vi "UHR-Fleezers Control (host) -TL FB Corrected Ronen.vi"(0 "Tab Control":T5(tab)=enum."DAQ AI") -> ()   [LabVIEW 2013] (continued)
                    }
                  }
                }
                event Mouse Up {
                  n1349 = event-data() -> ("Button"=w2095:u16)  [unwired: 8 out]
                  n1350 = case shown="3" w2095 {
                    tunnel: [FALSE TRUE] -> w2096
                    frame 0, Default {
                    }
                    frame 3 {
                      n1351 = local write "Manipulating Trap"(FALSE ("Manipulating Trap")) -> ()
                    }
                  }
                }
              }
            }
          }
        }
      }
      event Mouse Move {
        n1352 = event-data() -> ()  [unwired: 6 out]
      }
    }
    n1353 = local read "Stop All"() -> (w1917:bool)
    n1354 = node-c288() -> ()  [unwired: 2 out]
  }
  n1355 = node-c288(w34) -> ()  [unwired: 1 out]
  n1356 = node-c288(w88) -> ()  [unwired: 1 out]
  n1357 = node-c288(w95) -> ()  [unwired: 1 out]
  n1358 = node-c288(i64 1 ("Period"), 1 ("Processor")) -> (w182:T25)  [unwired: 2 out]
  n1359 = timed-loop "Acquire Data" {
    tunnel: w44 -> [w2380]
    tunnel: w60 -> [w2379]
    tunnel: [w2410] -> w53
    tunnel: [w2404] -> w52
    timing: w182 -> [_]
    timing-out: [_] -> w181
    tunnel: w79 -> [w2215]
    stop <- "Stop All" stop-if-true
    (unwired) u32 0 ("Number of Elements")
    w2202 = "NI_ChannelName" ("name")
    n1360 = node-c288() -> ()  [unwired: 2 out]
    n1361 = First Call?() -> (First Call?: T/F=w2168:bool)
    n1362 = Or(x="Reset", y=w2168) -> (x .or. y?=w2169:bool)
    n1363 = local read "MCL Tracking"() -> (w2105:bool)
    n1364 = case "Reset data stream" shown="True" w2169 {
      tunnel: w2380 -> [w2478 w2486]
      tunnel: w2379 -> [w2477 w2485]
      tunnel: [w2478 w2480] -> w2103
      tunnel: [w2477 w2479] -> w2375
      frame False {
      }
      frame True {
        w2483 = TRUE ("AI to FIFO")
        n1365 = local write "Overflow (data lost)"(FALSE ("Overflow (data lost)")) -> ()
        n1366 = call "reset FPGA DMA.vi"("error in"=w2485, "FPGA VI Reference In"=w2486) -> ("error out"=w2481:errorcluster, "FPGA VI Reference Out"=w2482:T20)
        n1367 = xnode "Read/Write Control"("FPGA VI Reference In"=w2482, "error in"=w2481, "AI to FIFO"=w2483, "APD to FIFO"=w2483) -> ("FPGA VI Reference Out"=w2480:T20, "error out"=w2479:errorcluster)
      }
    }
    n1368 = Or(x="Start AOD Scan", y="Trap Raster Scan") -> (x .or. y?=w2331:bool)
    n1369 = case "Start AOM raster scan" shown="True" w2331 {
      tunnel: w2103 -> [w3215 w3225]
      tunnel: w2375 -> [w3214 w3224]
      tunnel: [w3215 w3218] -> w2102
      tunnel: [w3214 w3217] -> w2374
      frame False {
      }
      frame True {
        n1370 = case shown="True" "Restart DMA? (AOD)" {
          tunnel: [w3263 w3265] -> w3219
          tunnel: [w3262 w3264] -> w3220
          tunnel: w3225 -> [w3263 w3267]
          tunnel: w3224 -> [w3262 w3266]
          frame False {
          }
          frame True {
            n1371 = local write "Overflow (data lost)"(FALSE ("Overflow (data lost)")) -> ()
            n1372 = call "reset FPGA DMA.vi"("error in"=w3266, "FPGA VI Reference In"=w3267) -> ("error out"=w3264:errorcluster, "FPGA VI Reference Out"=w3265:T20)
          }
        }
        n1373 = local write "Trap Raster Scan"(FALSE ("Trap Raster Scan")) -> ()
        n1374 = case shown="True" "Move MCL Also?" {
          tunnel: w3220 -> [w3228 w3257]
          tunnel: w3219 -> [w3229 w3258]
          tunnel: [w3227 w3261] -> w3218
          tunnel: [w3226 w3260] -> w3217
          frame False {
            w3230 = TRUE ("AI to FIFO")
            n1375 = xnode "Read/Write Control"("FPGA VI Reference In"=w3229, "error in"=w3228, "AI to FIFO"=w3230, "APD to FIFO"=w3230, "Start scan"=w3230) -> ("FPGA VI Reference Out"=w3227:T20, "error out"=w3226:errorcluster)
          }
          frame True {
            w3254 = FALSE ("1D or 2D Scan?")
            w3259 = TRUE ("AI to FIFO")
            # "Count for MCL loop"
            # "N total cycles"
            # "N steps"
            # "V_int"
            n1376 = local read "Scan Range (nm)"() -> (w3236:dbl)
            n1377 = local read "Number of F/B Scans (AOD)"() -> (w3253:u16)
            n1378 = Sign(1:w3236) -> (0:w3235:dbl)
            n1379 = Compound Arithmetic op=MULTIPLY(w3236, "MCL Step Position Ratio", "MCL/AOM Scale Tweak") -> (w3240:dbl)
            n1380 = Negate(x=w3235) -> (-x=w3232:dbl)
            n1381 = Multiply(x=w3232, y="MCL Step Increment (V_int)") -> (x*y=w3234:dbl)
            n1382 = Divide(x=w3240, y="MCL X Cal (nm/V)") -> (x/y=w3246:dbl)
            n1383 = Multiply(x=32767.0 ("y"), y=w3246) -> (x*y=w3252:dbl)
            n1384 = local read "Total Counts (ticks)"() -> (w3237:u32)
            n1385 = local read "Cycles/step (AOD)"() -> (w3248:u64)
            n1386 = local read "Scan steps (AOD)"() -> (w3249:u64)
            n1387 = Divide(x=w3252, y=10.0) -> (x/y=w3245:dbl)
            n1388 = Divide(x=w3245, y="MCL Step Increment (V_int)") -> (x/y=w3243:dbl)
            n1389 = Absolute Value(x=w3243) -> (abs(x)=w3231:dbl)
            n1390 = Compound Arithmetic op=MULTIPLY(w3249, w3248, w3237) -> (w3244:u64)
            n1391 = local write "wait to reset values"(w3259) -> ()
            n1392 = local write "MCL Scanning"(w3259) -> ()
            n1393 = Divide(x=w3244, y=w3231) -> (x/y=w3241:dbl)
            "MCL Count" <- w3241
            n1394 = xnode "Read/Write Control"("FPGA VI Reference In"=w3258, "error in"=w3257, "Scan steps (MCL)"=w3231, "Number of scans (MCL)"=w3253, "Cycles per step (MCL)"=u64 1, "Scan freq.  increment (MCL)"=w3234, "1D or 2D Scan?"=w3254, "MCL Scan Axis"=w3254, "Cont. Scan (MCL)"=w3254, "MCL count"=w3241) -> ("FPGA VI Reference Out"=w3256:T20, "error out"=w3255:errorcluster)
            n1395 = xnode "Read/Write Control"("FPGA VI Reference In"=w3256, "error in"=w3255, "AI to FIFO"=w3259, "APD to FIFO"=w3259, "Start scan"=w3259, "Start scan (MCL)"=w3259) -> ("FPGA VI Reference Out"=w3261:T20, "error out"=w3260:errorcluster)
          }
        }
        "Raster Scanning..." <- TRUE ("Scanning...")
      }
    }
    n1396 = And(x="Save scans", y=w2331) -> (x .and. y?=w2373:bool)
    n1397 = Compound Arithmetic op=OR("Start MCL Scan", "Confocal Image", "Confocal Linescan") -> (w2329:bool)
    n1398 = And(x="Save Data (MCL)", y=w2329) -> (x .and. y?=w2372:bool)
    n1399 = case "Start MCL raster scan" shown="True" w2329 {
      tunnel: w2102 -> [w2769 w2784]
      tunnel: w2374 -> [w2768 w2783]
      tunnel: [w2769 w2779] -> w2138
      tunnel: [w2768 w2778] -> w2137
      tunnel: [FALSE w2777] -> w2358
      tunnel: "Start MCL Scan" -> [_ w2772]
      tunnel: "Confocal Image" -> [_ w2771]
      tunnel: "Confocal Linescan" -> [_ _]
      frame False {
      }
      frame True {
        w2777 = TRUE
        n1400 = case shown="True" "Restart DMA? (MCL)" {
          tunnel: [w2829 w2831] -> w2782
          tunnel: [w2828 w2830] -> w2781
          tunnel: w2784 -> [w2829 w2834]
          tunnel: w2783 -> [w2828 w2833]
          frame False {
          }
          frame True {
            n1401 = call "reset FPGA DMA.vi"("error in"=w2833, "FPGA VI Reference In"=w2834) -> ("error out"=w2830:errorcluster, "FPGA VI Reference Out"=w2831:T20)
            n1402 = local write "Overflow (data lost)"(FALSE ("Overflow (data lost)")) -> ()
          }
        }
        n1403 = case shown="False" w2772 {
          selector: w2772 -> [_ w2788]
          tunnel: w2771 -> [w2787 _]
          tunnel: [w2787 w2788] -> w2770
          frame False {
            n1404 = property on="2D or 1D Scan" class="Bool (strict)"("Val(Sgnl)"=w2787) -> ()  [unwired: 2 in, 2 out]
            n1405 = property on="Confocal Image" class="Bool (strict)"("Value"=FALSE ("Start Confocal Map")) -> ()  [unwired: 2 in, 2 out]
          }
          frame True {
          }
        }
        n1406 = local write "MCL Scanning"(w2777) -> ()
        n1407 = local read "AO1"() -> (w2774:dbl)
        n1408 = local read "AO2"() -> (w2773:dbl)
        n1409 = case shown="True" "Center Scan" {
          tunnel: w2782 -> [w2795 w2827]
          tunnel: w2781 -> [w2794 w2826]
          tunnel: [w2793 w2825] -> w2779
          tunnel: [w2792 w2824] -> w2778
          tunnel: [w2790 w2811] -> w2776
          tunnel: [w2789 w2810] -> w2775
          tunnel: w2774 -> [w2790 w2816]
          tunnel: w2773 -> [w2789 w2819]
          tunnel: w2770 -> [_ _]
          frame False {
            w2791 = TRUE ("AI to FIFO")
            n1410 = xnode "Read/Write Control"("FPGA VI Reference In"=w2795, "error in"=w2794, "AI to FIFO"=w2791, "APD to FIFO"=w2791, "Start scan (MCL)"=w2791) -> ("FPGA VI Reference Out"=w2793:T20, "error out"=w2792:errorcluster)
          }
          frame True {
            w2823 = TRUE ("AI to FIFO")
            n1411 = local read "Scan steps (MCL)"() -> (w2802:u64)
            n1412 = local read "Scan lines (y)"() -> (w2798:u64)
            n1413 = local read "Fast Scan Dir"() -> (w2809:bool)
            n1414 = local read "Actual MCL Inc (V)"() -> (w2799:dbl)
            n1415 = Decrement(x=w2798) -> (x-1=w2797:u64)
            n1416 = Decrement(x=w2802) -> (x-1=w2801:u64)
            n1417 = Multiply(x=w2799, y=w2797) -> (x*y=w2796:dbl)
            n1418 = Divide(x=w2796, y=2.0) -> (x/y=w2806:dbl)
            n1419 = Multiply(x=w2799, y=w2801) -> (x*y=w2800:dbl)
            n1420 = Divide(x=w2800, y=2.0) -> (x/y=w2805:dbl)
            n1421 = Select(t=w2805, s=w2809, f=w2806) -> (s? t:f=w2804:dbl)
            n1422 = Select(t=w2806, s=w2809, f=w2805) -> (s? t:f=w2808:dbl)
            n1423 = Subtract(x=w2816, y=w2808) -> (x-y=w2807:dbl)
            n1424 = Subtract(x=w2819, y=w2804) -> (x-y=w2803:dbl)
            n1425 = local read "2D or 1D Scan"() -> (w2821:bool)
            n1426 = Not(x=w2809) -> (.not. x?=w2815:bool)
            n1427 = Not(x=w2821) -> (.not. x?=w2817:bool)
            n1428 = And(x=w2809, y=w2817) -> (x .and. y?=w2818:bool)
            n1429 = And(x=w2817, y=w2815) -> (x .and. y?=w2820:bool)
            n1430 = Select(t=w2819, s=w2820, f=w2803) -> (s? t:f=w2810:dbl)
            n1431 = Select(t=w2816, s=w2818, f=w2807) -> (s? t:f=w2811:dbl)
            n1432 = call "Volt to I16.vi"("Voltage In"=w2811) -> ("I16 Voltage Out"=w2814:i16)
            n1433 = call "Volt to I16.vi"("Voltage In"=w2810) -> ("I16 Voltage Out"=w2813:i16)
            n1434 = xnode "Read/Write Control"("FPGA VI Reference In"=w2827, "error in"=w2826, "AI to FIFO"=w2823, "APD to FIFO"=w2823, "Start scan (MCL)"=w2823, "AO1"=w2814, "AO2"=w2813) -> ("FPGA VI Reference Out"=w2825:T20, "error out"=w2824:errorcluster)
          }
        }
        "Initial Y" <- w2776
        "Initial X" <- w2775
        "wait to reset values" <- w2777
      }
    }
    n1435 = local read "Trap Pos Elements/DMA read"() -> (w2211:u32)
    n1436 = local read "Trap AI Elements/DMA read"() -> (w2136:u32)
    n1437 = local read "APD Elements/DMA read"() -> (w2254:u32)
    n1438 = local read "Trap AI FIFO Depth"() -> (w2420:u32)
    n1439 = xnode "Invoke Method"("FPGA VI Reference In"=w2138, "error in"=w2137, "Number of Elements"=w2211, "Timeout (ms)"=-1) -> ("Data"=w2175:u16[], "Elements Remaining"=→"Trap Pos FIFO El Remaining":u32)  [unwired: 2 out]
    n1440 = xnode "Invoke Method"("FPGA VI Reference In"=w2138, "error in"=w2137, "Number of Elements"=w2136, "Timeout (ms)"=-1 ("Timeout")) -> ("FPGA VI Reference Out"=w2107:T20, "error out"=w2139:errorcluster, "Data"=w2135:i16[], "Elements Remaining"=w2140:u32)
    "Trap AI FIFO El. Rem." <- w2140
    n1441 = xnode "Get APD Data"("FPGA VI Reference In"=w2138, "error in"=w2137, "Number of Elements"=w2254, "Timeout (ms)"=-1) -> ("Data"=w2253:u32[], "Elements Remaining"=→"APD FIFO Elements Remaining":u32)  [unwired: 2 out]
    n1442 = Subtract(x=w2420, y=w2136) -> (x-y=w2419:u32)
    n1443 = Decimate 1D Array(w2175) -> (w2172:u16[], w2174:u16[], w2173:u16[])
    n1444 = Divide(x=w2140, y=w2419) -> (x/y=w2418:dbl)
    "Buffer Status" <- w2418
    n1445 = To Unsigned Long Integer(number=w2172) -> (unsigned 32bit integer=w2171:u32[])
    n1446 = Join Numbers(hi=w2174, lo=w2173) -> ((hi.lo)=w2170:u32[])
    n1447 = Equal?(x=w2418, y=1.0) -> (x = y?=w2416:bool)
    n1448 = Join Numbers(hi=w2171, lo=w2170) -> ((hi.lo)=w2164:u64[])
    n1449 = call "IR AOM word to freq - vec.vi"("Frequency Word In (double vec)"=w2164) -> ("Frequency Out"=w2210:dbl[])
    n1450 = case "Alert buffer overflow" shown="False" w2416 {
      frame False {
      }
      frame True {
        n1451 = call <vilib>:"Beep.vi"() -> ()  [unwired: 3 in, 9 out]
        "Overflow (data lost)" <- TRUE ("Overflow (data lost)")
      }
    }
    n1452 = Decimate 1D Array(w2210) -> (w2209:dbl[], w2208:dbl[])
    n1453 = Array Size(array=w2135) -> (size(s)=→"Waveform Chart":i32)
    n1454 = Build Array(w2209, w2208) -> (w2207:dbl[][])
    n1455 = local read "Trap Sets"() -> (w2291:u32)
    n1456 = case "Deinterlace trap data, average down PSD" shown="2" w2291 {
      tunnel: w2135 -> [w2864 w2929]
      tunnel: [w2861 w2926] -> w2284
      tunnel: [w2864 w2928] -> w2167
      tunnel: "Detector Type" -> [w2863 w2924]
      tunnel: [w2862 w2927] -> w2283
      tunnel: [w2860 w2925] -> w2391
      frame 1, Default {
        n1457 = Divide(x=w2864, y=3276.7) -> (x/y=w2865:dbl[])
        n1458 = Decimate 1D Array(w2865) -> (w2874:dbl[], w2873:dbl[], w2872:dbl[], w2871:dbl[], w2870:dbl[], w2869:dbl[], w2868:dbl[], w2867:dbl[])
        n1459 = case shown="\"IR-QPD + PSD + FB-QPD position\"" w2863 {
          tunnel: w2874 -> [w2898 w2923]
          tunnel: w2873 -> [w2897 w2922]
          tunnel: w2872 -> [w2882 w2900]
          tunnel: w2871 -> [w2883 w2910]
          tunnel: w2870 -> [w2896 w2921]
          tunnel: w2869 -> [w2895 w2920]
          tunnel: w2868 -> [w2879 w2901]
          tunnel: w2867 -> [w2878 w2899]
          tunnel: [w2877 w2907] -> w2862
          tunnel: [w2876 w2906] -> w2861
          tunnel: [w2875 w2905] -> w2860
          frame "IR-QPD + PSD + FB-QPD", Default {
            w2875 = 0  # Channel pattern
            n1460 = Divide(x=w2898, y=w2883) -> (x/y=w2885:dbl[])
            n1461 = Divide(x=w2897, y=w2883) -> (x/y=w2884:dbl[])
            n1462 = Divide(x=w2896, y=w2879) -> (x/y=w2881:dbl[])
            n1463 = Divide(x=w2895, y=w2878) -> (x/y=w2880:dbl[])
            n1464 = Build Array(w2885, w2884, w2883, w2882, w2881, w2880, w2879, w2878) -> (w2876:dbl[][])
            n1465 = Bundle("T1 Y", "T1 X", "T1 Sum", "FB Sum", "PSD Y", "PSD X", "PSD Y Sum", "PSD X Sum") -> (w2894:T42)  [unwired: 1 out]
            n1466 = Cluster To Array(cluster=w2894) -> (array=w2877:string[])
          }
          frame "IR-QPD + PSD + FB-QPD position" {
            w2905 = 3  # Channel pattern
            n1467 = Negate(x=w2901) -> (-x=w2902:dbl[])
            n1468 = Divide(x=w2923, y=w2910) -> (x/y=w2912:dbl[])
            n1469 = Divide(x=w2922, y=w2910) -> (x/y=w2911:dbl[])
            n1470 = Divide(x=w2921, y=w2901) -> (x/y=w2909:dbl[])
            n1471 = Divide(x=w2920, y=w2902) -> (x/y=w2908:dbl[])
            n1472 = Build Array(w2912, w2911, w2910, w2899, w2900, w2909, w2908, w2901) -> (w2906:dbl[][])
            n1473 = Bundle("T1 Y", "T1 X", "T1 Sum", "FB X", "FB Sum", "PSD Y", "PSD X", "PSD Y Sum") -> (w2919:T42)  [unwired: 1 out]
            n1474 = Cluster To Array(cluster=w2919) -> (array=w2907:string[])
          }
        }
      }
      frame 2 {
        n1475 = case shown="\"UCB Fleezers 052511\"" w2924 {
          tunnel: w2929 -> [w2991 w3058 w3086 w3193]
          tunnel: [w2930 w3050 w3081 w3124] -> w2928
          tunnel: [w2957 w3041 w3083 w3171] -> w2927
          tunnel: [w2956 w3005 w3060 w3138] -> w2926
          tunnel: [w2950 w3040 w3123 w3169] -> w2925
          frame "IR-QPD + PSD + FB-QPD", Default {
            w2950 = 1  # Channel pattern
            # "time average x2 the 4th signal and the 4 psd signals (detection laser)"
            # "deinterlace 3 signals from qpd"
            n1476 = Decimate 1D Array(w2991) -> (w2990:i16[], w2989:i16[], w2955:i16[], w2988:i16[], w2978:i16[], w2976:i16[], w2975:i16[], w2973:i16[])
            n1477 = call "downsample 1D array - double.vi"("Ave N"=2.0, "Array In"=w2978) -> ("Array Out"=w2977:dbl[])  [unwired: 1 out]
            n1478 = call "downsample 1D array - double.vi"("Ave N"=2.0, "Array In"=w2973) -> ("Array Out"=w2972:dbl[])  [unwired: 1 out]
            n1479 = call "downsample 1D array - double.vi"("Ave N"=2.0, "Array In"=w2975) -> ("Array Out"=w2974:dbl[])  [unwired: 1 out]
            n1480 = call "downsample 1D array - double.vi"("Ave N"=2.0, "Array In"=w2976) -> ("Array Out"=w2958:dbl[])  [unwired: 1 out]
            n1481 = Decimate 1D Array(w2990) -> (w2987:i16[], w2959:i16[])
            n1482 = Decimate 1D Array(w2989) -> (w2986:i16[], w2984:i16[])
            n1483 = Decimate 1D Array(w2988) -> (w2985:i16[], w2983:i16[])
            n1484 = Decimate 1D Array(w2955) -> (w2954:i16[], w2953:i16[])
            n1485 = Interleave 1D Arrays(w2987, w2986, w2985, w2959, w2984, w2983, w2954, w2953, w2977, w2958, w2974, w2972) -> (w2971:dbl[])
            n1486 = To Word Integer(number=w2971) -> (16bit integer=w2930:i16[])
            n1487 = Divide(x=w2971, y=3276.7) -> (x/y=w2970:dbl[])
            n1488 = Decimate 1D Array(w2970) -> (w2969:dbl[], w2968:dbl[], w2967:dbl[], w2966:dbl[], w2965:dbl[], w2964:dbl[], w2952:dbl[], w2951:dbl[], w2963:dbl[], w2962:dbl[], w2961:dbl[], w2960:dbl[])
            n1489 = Divide(x=w2969, y=w2967) -> (x/y=w2937:dbl[])
            n1490 = Divide(x=w2968, y=w2967) -> (x/y=w2936:dbl[])
            n1491 = Divide(x=w2966, y=w2964) -> (x/y=w2935:dbl[])
            n1492 = Divide(x=w2965, y=w2964) -> (x/y=w2934:dbl[])
            n1493 = Divide(x=w2963, y=w2961) -> (x/y=w2933:dbl[])
            n1494 = Divide(x=w2962, y=w2960) -> (x/y=w2932:dbl[])
            n1495 = Bundle("T1 Y", "T1 X", "T1 Sum", "T2 Y", "T2 X", "T2 Sum", "T1 FB Sum", "T2 FB Sum", "PSD Y", "PSD X", "PSD Y Sum", "PSD X Sum") -> (w2938:T43)  [unwired: 1 out]
            n1496 = Build Array(w2937, w2936, w2967, w2935, w2934, w2964, w2952, w2951, w2933, w2932, w2961, w2960) -> (w2956:dbl[][])
            n1497 = Cluster To Array(cluster=w2938) -> (array=w2957:string[])
          }
          frame "IR-QPD + PSD + FB-QPD X position" {
            w3040 = 2  # Channel pattern
            # "convert\nADC numbers\nto volts"
            # "time average x2 the 3 psd signals (detection laser)"
            # "deinterlace 3 signals from qpds"
            n1498 = Decimate 1D Array(w3058) -> (w3057:i16[], w3056:i16[], w2993:i16[], w2994:i16[], w3003:i16[], w3000:i16[], w2997:i16[], w3028:i16[])
            n1499 = Decimate 1D Array(w3057) -> (w3055:i16[], w3042:i16[])
            n1500 = call "downsample 1D array - I16.vi"("Ave N"=2.0, "Array In"=w3003) -> ("Array Out"=w3001:i16[])  [unwired: 1 in]
            n1501 = call "downsample 1D array - I16.vi"("Ave N"=2.0, "Array In"=w3000) -> ("Array Out"=w2998:i16[])  [unwired: 1 in]
            n1502 = Decimate 1D Array(w3056) -> (w3054:i16[], w3052:i16[])
            n1503 = Decimate 1D Array(w2994) -> (w3053:i16[], w3051:i16[])
            n1504 = Decimate 1D Array(w3028) -> (w3027:i16[], w3025:i16[])
            n1505 = Decimate 1D Array(w2993) -> (w3026:i16[], w3024:i16[])
            n1506 = call "downsample 1D array - I16.vi"("Ave N"=2.0, "Array In"=w2997) -> ("Array Out"=w2995:i16[])  [unwired: 1 in]
            n1507 = Interleave 1D Arrays(w3055, w3054, w3053, w3042, w3052, w3051, w3027, w3026, w3025, w3024, w3001, w2998, w2995) -> (w3050:i16[])
            n1508 = Divide(x=w3050, y=3276.7) -> (x/y=w3049:dbl[])
            n1509 = Decimate 1D Array(w3049) -> (w3048:dbl[], w3047:dbl[], w3046:dbl[], w3045:dbl[], w3044:dbl[], w3043:dbl[], w3016:dbl[], w3014:dbl[], w3013:dbl[], w3011:dbl[], w3010:dbl[], w3009:dbl[], w3006:dbl[])
            n1510 = Divide(x=w3048, y=w3046) -> (x/y=w3032:dbl[])
            n1511 = Divide(x=w3047, y=w3046) -> (x/y=w3031:dbl[])
            n1512 = Divide(x=w3045, y=w3043) -> (x/y=w3030:dbl[])
            n1513 = Divide(x=w3044, y=w3043) -> (x/y=w3029:dbl[])
            n1514 = Divide(x=w3016, y=w3014) -> (x/y=w3015:dbl[])
            n1515 = Divide(x=w3013, y=w3011) -> (x/y=w3012:dbl[])
            n1516 = Divide(x=w3010, y=w3006) -> (x/y=w3008:dbl[])
            n1517 = Negate(x=w3006) -> (-x=w3004:dbl[])
            n1518 = Divide(x=w3009, y=w3004) -> (x/y=w3007:dbl[])
            n1519 = Bundle("T1 Y", "T1 X", "T1 Sum", "T2 Y", "T2 X", "T2 Sum", "T1 FB X", "T1 FB Sum", "T2 FB X", "T2 FB Sum", "PSD Y", "PSD X", "PSD Y Sum") -> (w3033:T44)  [unwired: 1 out]
            n1520 = Build Array(w3032, w3031, w3046, w3030, w3029, w3043, w3015, w3014, w3012, w3011, w3008, w3007, w3006) -> (w3005:dbl[][])
            n1521 = Cluster To Array(cluster=w3033) -> (array=w3041:string[])
          }
          frame "UCB Fleezers 052511" {
            w3123 = 2  # Channel pattern
            n1522 = Decimate 1D Array(w3086) -> (w3121:i16[], w3120:i16[], w3085:i16[], w3084:i16[], w3078:i16[], w3075:i16[], w3074:i16[], w3073:i16[])
            n1523 = Decimate 1D Array(w3121) -> (w3119:i16[], w3104:i16[])
            n1524 = Decimate 1D Array(w3120) -> (w3118:i16[], w3116:i16[])
            n1525 = Decimate 1D Array(w3085) -> (w3117:i16[], w3115:i16[])
            n1526 = Decimate 1D Array(w3084) -> (w3080:i16[], w3079:i16[])
            n1527 = Decimate 1D Array(w3078) -> (w3077:i16[], w3076:i16[])
            n1528 = call "downsample 1D array - I16.vi"("Ave N"=2.0, "Array In"=w3075) -> ("Array Out"=w3072:i16[])  [unwired: 1 in]
            n1529 = call "downsample 1D array - I16.vi"("Ave N"=2.0, "Array In"=w3074) -> ("Array Out"=w3071:i16[])  [unwired: 1 in]
            n1530 = call "downsample 1D array - I16.vi"("Ave N"=2.0, "Array In"=w3073) -> ("Array Out"=w3070:i16[])  [unwired: 1 in]
            n1531 = Interleave 1D Arrays(w3119, w3118, w3117, w3104, w3116, w3115, w3080, w3077, w3079, w3076, w3072, w3071, w3070) -> (w3081:i16[])
            n1532 = Divide(x=w3081, y=3276.7) -> (x/y=w3111:dbl[])
            n1533 = Decimate 1D Array(w3111) -> (w3110:dbl[], w3109:dbl[], w3108:dbl[], w3107:dbl[], w3106:dbl[], w3105:dbl[], w3069:dbl[], w3067:dbl[], w3066:dbl[], w3064:dbl[], w3063:dbl[], w3062:dbl[], w3061:dbl[])
            n1534 = Divide(x=w3110, y=w3108) -> (x/y=w3091:dbl[])
            n1535 = Divide(x=w3109, y=w3108) -> (x/y=w3090:dbl[])
            n1536 = Divide(x=w3107, y=w3105) -> (x/y=w3089:dbl[])
            n1537 = Divide(x=w3106, y=w3105) -> (x/y=w3088:dbl[])
            n1538 = Divide(x=w3069, y=w3067) -> (x/y=w3068:dbl[])
            n1539 = Divide(x=w3066, y=w3064) -> (x/y=w3065:dbl[])
            n1540 = Bundle("T1 Y", "T1 X", "T1 Sum", "T2 Y", "T2 X", "T2 Sum", "T1 FB X", "T2 FB Sum", "T2 FB X", "T2 FB Sum", "PSD Y", "PSD X", "PSD Sum") -> (w3092:T44)  [unwired: 1 out]
            n1541 = Build Array(w3091, w3090, w3108, w3089, w3088, w3105, w3068, w3067, w3065, w3064, w3063, w3062, w3061) -> (w3060:dbl[][])
            n1542 = Cluster To Array(cluster=w3092) -> (array=w3083:string[])
          }
          frame "IR-QPD + PSD + FB-QPD XY positions" {
            w3169 = 4  # Channel pattern
            # "time average x2 the 3 psd signals (detection laser)"
            # "deinterlace 3 signals from qpds"
            n1543 = Decimate 1D Array(w3193) -> (w3192:i16[], w3191:i16[], w3170:i16[], w3190:i16[], w3136:i16[], w3182:i16[], w3181:i16[], w3158:i16[])
            n1544 = Decimate 1D Array "QPD Y"(w3192) -> (w3189:i16[], w3172:i16[])
            n1545 = call "downsample 1D array - double.vi"("Ave N"=2.0, "Array In"=w3182) -> ("Array Out"=w3157:dbl[])  [unwired: 1 out]
            n1546 = call "downsample 1D array - double.vi"("Ave N"=2.0, "Array In"=w3181) -> ("Array Out"=w3156:dbl[])  [unwired: 1 out]
            n1547 = Decimate 1D Array "Feedback Sum"(w3170) -> (w3154:i16[], w3152:i16[])
            n1548 = Decimate 1D Array "Feedback Y"(w3136) -> (w3135:i16[], w3134:i16[])
            n1549 = Decimate 1D Array "Feedback X"(w3158) -> (w3155:i16[], w3153:i16[])
            n1550 = Decimate 1D Array "QPD Sum"(w3190) -> (w3187:i16[], w3185:i16[])
            n1551 = Decimate 1D Array "QPD X"(w3191) -> (w3188:i16[], w3186:i16[])
            n1552 = Interleave 1D Arrays(w3189, w3188, w3187, w3172, w3186, w3185, w3135, w3155, w3154, w3134, w3153, w3152, w3157, w3156) -> (w3180:dbl[])
            n1553 = To Word Integer(number=w3180) -> (16bit integer=w3124:i16[])
            n1554 = Divide(x=w3180, y=3276.7) -> (x/y=w3179:dbl[])
            n1555 = Decimate 1D Array(w3179) -> (w3178:dbl[], w3177:dbl[], w3176:dbl[], w3175:dbl[], w3174:dbl[], w3173:dbl[], w3131:dbl[], w3145:dbl[], w3129:dbl[], w3130:dbl[], w3143:dbl[], w3127:dbl[], w3141:dbl[], w3139:dbl[])
            n1556 = Divide(x=w3178, y=w3176) -> (x/y=w3162:dbl[])
            n1557 = Divide(x=w3177, y=w3176) -> (x/y=w3161:dbl[])
            n1558 = Divide(x=w3175, y=w3173) -> (x/y=w3160:dbl[])
            n1559 = Divide(x=w3174, y=w3173) -> (x/y=w3159:dbl[])
            n1560 = Divide(x=w3131, y=w3129) -> (x/y=w3128:dbl[])
            n1561 = Divide(x=w3145, y=w3129) -> (x/y=w3144:dbl[])
            n1562 = Divide(x=w3130, y=w3127) -> (x/y=w3126:dbl[])
            n1563 = Divide(x=w3143, y=w3127) -> (x/y=w3142:dbl[])
            n1564 = Negate(x=w3139) -> (-x=w3137:dbl[])
            n1565 = Divide(x=w3141, y=w3137) -> (x/y=w3140:dbl[])
            n1566 = Bundle("T1 Y", "T1 X", "T1 Sum", "T2 Y", "T2 X", "T2 Sum", "T1 FB Y", "T1 FB X", "T1 FB Sum", "T2 FB Y", "T2 FB X", "T2 FB Sum", "PSD X", "PSD Y Sum") -> (w3125:T45)  [unwired: 1 out]
            n1567 = Build Array(w3162, w3161, w3176, w3160, w3159, w3173, w3128, w3144, w3129, w3126, w3142, w3127, w3140, w3139) -> (w3138:dbl[][])
            n1568 = Cluster To Array(cluster=w3125) -> (array=w3171:string[])
          }
        }
      }
    }
    "AI labels" <- w2283
    n1569 = xnode "Read/Write Control"("FPGA VI Reference In"=w2107) -> ("FPGA VI Reference Out"=w2106:T20, "BD1 Frequency Out 1"=w2121:u64)  [unwired: 1 in, 1 out]
    n1570 = local read "BD 1 Frequency 2 (MHz)"() -> (w2112:dbl)
    n1571 = To Double Precision Float(number=w2121) -> (double precision float=w2118:dbl)
    n1572 = Multiply(x=49125000.0, y=6.0) -> (x*y=w2117:dbl)
    n1573 = Multiply(x=w2118, y=w2117) -> (x*y=w2115:dbl)
    n1574 = Scale By Power Of 2(n=-48, x=w2115) -> (x*2^n=w2114:dbl)
    n1575 = local read "Dynamic Force FB"() -> (w2111:bool)
    n1576 = local read "Trap Pos. FB ON"() -> (w2110:bool)
    n1577 = Divide(x=w2114, y=1000000.0) -> (x/y=w2104:dbl)
    n1578 = case shown="True" w2105 {
      tunnel: w2104 -> [_ w2454]
      tunnel: w2102 -> [_ w2441]
      frame False {
      }
      frame True {
        n1579 = local read "AOM X Cal (nm/MHz)"() -> (w2451:dbl)
        n1580 = local read "Zero T1 position"() -> (w2453:dbl)
        n1581 = Subtract(x=w2454, y=w2453) -> (x-y=w2452:dbl)
        n1582 = Multiply(x=w2452, y=w2451) -> (x*y=w2450:dbl)
        n1583 = local read "MCL X Cal (nm/V)"() -> (w2447:dbl)
        n1584 = Multiply(x=w2450, y="Tracking factor") -> (x*y=w2448:dbl)
        n1585 = local read "Zero MCL x position"() -> (w2446:dbl)
        n1586 = Divide(x=w2448, y=w2447) -> (x/y=w2445:dbl)
        n1587 = Add(x=w2446, y=w2445) -> (x+y=w2438:dbl)
        "Current MCL (V)" <- w2438
        n1588 = Multiply(x=w2438, y=32767.0) -> (x*y=w2442:dbl)
        n1589 = Divide(x=w2442, y=10.0) -> (x/y=w2439:dbl)
        n1590 = To Word Integer(number=w2439) -> (16bit integer=w2440:i16)
        n1591 = xnode "Read/Write Control"("FPGA VI Reference In"=w2441, "AO2"=w2440) -> ()  [unwired: 1 in, 2 out]
      }
    }
    n1592 = Subtract(x=w2112, y=w2104) -> (x-y=w2100:dbl)
    "Current deltaFreq" <- w2100
    n1593 = Compound Arithmetic op=AND(w2111, w2110, "Real time offset \ncorrection for setpoint") -> (w2108:bool)
    n1594 = case shown="True" w2108 {
      tunnel: w2100 -> [_ w2455]
      frame False {
      }
      frame True {
        n1595 = local read "T1 kappa_x (pN/nm)"() -> (w2464:dbl)
        n1596 = local read "T1 alpha_x (nm/V)"() -> (w2465:dbl)
        n1597 = local read "Negate offset difference"() -> (w2466:bool)
        n1598 = local read "Offset file step size"() -> (w2474:dbl)
        n1599 = Multiply(x="Target Force (pN)", y=2.0) -> (x*y=w2462:dbl)
        n1600 = local read "Setpoint offset\nCorrection values"() -> (w2471:dbl[])
        n1601 = Divide(x=w2455, y=w2474) -> (x/y=w2473:dbl)
        n1602 = Select(t=-1, s=w2466, f=1) -> (s? t:f=w2467:i32)
        n1603 = To Long Integer(number=w2473) -> (32bit integer=w2472:i32)
        n1604 = Multiply(x=w2465, y=w2464) -> (x*y=w2461:dbl)
        n1605 = Divide(x=w2462, y=w2461) -> (x/y=w2460:dbl)
        n1606 = Index Array(array=w2471, index=w2472) -> (element=w2470:dbl)
        n1607 = Multiply(x=w2467, y=w2470) -> (x*y=w2459:dbl)
        n1608 = Add(x=w2460, y=w2459) -> (x+y=w2458:dbl)
        n1609 = To Fixed-Point(number=w2458) -> (fixed-point=w2457:fxp<+/-,16,1>)  [unwired: 1 in]
        n1610 = property on="Trap Pos FB SP" class="DigNum (strict)"("Val(Sgnl)"=w2457) -> ()  [unwired: 2 in, 2 out]
      }
    }
    n1611 = case shown="False" "Take full offset data for display" {
      tunnel: [w2424 w2430] -> w2308
      tunnel: [w2423 w2429] -> w2306
      tunnel: w2100 -> [_ w2436]
      frame False {
        n1612 = Divide(x="T2 offset_x (mV)", y=1000.0) -> (x/y=w2423:dbl)
        n1613 = Divide(x="T1 offset_x (mV)", y=1000.0) -> (x/y=w2424:dbl)
      }
      frame True {
        n1614 = local read "Offset Values"() -> (w2437:T14)
        n1615 = local read "Offset file step size"() -> (w2435:dbl)
        n1616 = Unbundle By Name(w2437) -> ("Trap 1X offset"=w2432:dbl[], "Trap 2X offset"=w2431:dbl[])
        n1617 = Divide(x=w2436, y=w2435) -> (x/y=w2434:dbl)
        n1618 = To Long Integer(number=w2434) -> (32bit integer=w2433:i32)
        n1619 = Index Array(array=w2432, index=w2433) -> (element=w2430:dbl)
        n1620 = Index Array(array=w2431, index=w2433) -> (element=w2429:dbl)
      }
    }
    n1621 = Decimate 1D Array(w2253) -> (w2281:u32[], w2217:u32[])
    n1622 = local read "DMA Update Period (s)"() -> (w2292:dbl)
    n1623 = local read "BD 1 Frequency 2 (MHz)"() -> (w2159:dbl)
    n1624 = local read "BD 1 Frequency 1 (MHz)"() -> (w2160:dbl)
    n1625 = Build Array(w2281, w2217) -> (w2355:u32[][])
    n1626 = local read "Data Period (s)"() -> (w2266:dbl)
    n1627 = Decimate 1D Array(w2167) -> (w2190:i16[], w2189:i16[], w2187:i16[], w2186:i16[])  [unwired: 9 out]
    n1628 = To Double Precision Float(number=w2355) -> (double precision float=w2356:dbl[][])
    n1629 = local read "APD Integration Time (s)"() -> (w2230:dbl)
    n1630 = Divide(x=w2190, y=w2189) -> (x/y=w2191:dbl[])
    n1631 = Divide(x=w2187, y=w2186) -> (x/y=w2188:dbl[])
    n1632 = feedback #1(0.0) -> (w2204:dbl)
    n1633 = Add(x=w2292, y=w2204) -> (x+y=w2393:dbl)
    n1634 = feedback-in #1(w2393) -> ()
    n1635 = local read "AOM X Cal (nm/MHz)"() -> (w2157:dbl)
    n1636 = To Time Stamp(1:w2204) -> (0:w2203:timestamp)
    n1637 = Split 1D Array(array=w2191, index="N El. to Ave.") -> (second subarray=w2194:dbl[])  [unwired: 1 out]
    n1638 = Split 1D Array(array=w2188, index="N El. to Ave.") -> (second subarray=w2193:dbl[])  [unwired: 1 out]
    n1639 = local read "Trap X AI1 (DMA)"() -> (w2192:T13)
    n1640 = Multiply(x=w2266, y="Trap Disp. Downsample") -> (x*y=w2205:dbl)
    "Display Period (s)" <- w2205
    n1641 = Bundle("BD 1 Frequency 1 (MHz)"=w2160, "BD 1 Frequency 2 (MHz)"=w2159) -> (w2161:T46)  [unwired: 1 out]
    n1642 = for "Trap AI" {
      tunnel: [w2859] -> w2387 mode=indexing
      tunnel: w2203 -> [w2849]
      tunnel: "Trap Disp. Downsample" -> [w2857]
      tunnel: w2284 -> [w2855] mode=indexing
      tunnel: w2266 -> [w2854]
      tunnel: w2283 -> [w2853] mode=indexing
      tunnel: w2202 -> [w2852]
      tunnel: [w2851] -> w2241 mode=indexing
      tunnel: w2205 -> [w2850]
      n1643 = Bundle By Name("Y"=w2855, "dt"=w2854) -> (w2856:waveform(dbl))  [unwired: 1 out]
      n1644 = Set Waveform Attribute(5:w2853, 6:w2852, 7:w2856) -> (3:w2851:waveform(dbl))  [unwired: 1 in, 2 out]
      n1645 = call "downsample 1D array - double.vi"("Ave N"=w2857, "Array In"=w2855) -> ("Array Out"=w2858:dbl[])  [unwired: 1 out]
      n1646 = Bundle By Name(cluster=w2851, "t0"=w2849, "Y"=w2858, "dt"=w2850) -> (w2859:waveform(dbl))
    }
    n1647 = call-poly <vilib>:"Mean.vi"("X"=w2193) -> ("mean"=w2181:dbl)  [unwired: 1 out]
    n1648 = call-poly <vilib>:"Mean.vi"("X"=w2194) -> ("mean"=w2182:dbl)  [unwired: 1 out]
    n1649 = Cluster To Array(cluster=w2161) -> (array=w2158:dbl[])
    n1650 = Reciprocal(x=w2205) -> (1/x=→"Trap Disp. Freq. (Hz)":dbl)
    n1651 = local read "Data points/scans (MCL)"() -> (w2367:dbl)
    n1652 = To Fixed-Point(number=w2181) -> (fixed-point=w2179:fxp<+/-,16,1>)  [unwired: 1 in]
    n1653 = To Fixed-Point(number=w2182) -> (fixed-point=w2180:fxp<+/-,16,1>)  [unwired: 1 in]
    n1654 = Bundle("Trap 1 Pos.", "Trap 2 Pos.") -> (w2201:cluster{string, string})  [unwired: 1 out]
    n1655 = Bundle By Name(cluster=w2192, "Set 1"=w2180, "Set 2"=w2179) -> (→"Trap X AI1 (DMA)":T13)
    n1656 = Cluster To Array(cluster=w2201) -> (array=w2198:string[])
    n1657 = for "Trap Position" {
      tunnel: w2207 -> [w2499] mode=indexing
      tunnel: "Trap Disp. Downsample" -> [w2498]
      tunnel: w2205 -> [w2496]
      tunnel: w2203 -> [w2495]
      tunnel: w2202 -> [w2493]
      tunnel: w2198 -> [w2492] mode=indexing
      tunnel: [w2491] -> w2156 mode=indexing
      tunnel: w2158 -> [w2489] mode=indexing
      tunnel: w2157 -> [w2487]
      n1658 = call "downsample 1D array - double.vi"("Ave N"=w2498, "Array In"=w2499) -> ("Array Out"=w2497:dbl[])  [unwired: 1 out]
      n1659 = Subtract(x=w2497, y=w2489) -> (x-y=w2490:dbl[])
      n1660 = Multiply(x=w2487, y=w2490) -> (x*y=w2488:dbl[])
      n1661 = Bundle By Name("Y"=w2488, "dt"=w2496, "t0"=w2495) -> (w2494:waveform(dbl))  [unwired: 1 out]
      n1662 = Set Waveform Attribute(5:w2492, 6:w2493, 7:w2494) -> (3:w2491:waveform(dbl))  [unwired: 1 in, 2 out]
    }
    "Trap Positions" <- w2156
    n1663 = Bundle("APD 1", "APD 2") -> (w2386:cluster{string, string})  [unwired: 1 out]
    n1664 = Cluster To Array(cluster=w2386) -> (array=w2383:string[])
    n1665 = for "APD" {
      tunnel: w2356 -> [w2838] mode=indexing
      tunnel: w2230 -> [w2846]
      tunnel: [w2842] -> w2237 mode=indexing
      tunnel: "APD Disp. Scale" -> [w2843]
      tunnel: w2202 -> [w2841]
      tunnel: w2383 -> [w2840] mode=indexing
      tunnel: "APD Disp. Downsample" -> [w2836]
      tunnel: [w2839] -> w2382
      tunnel: w2203 -> [w2835]
      n1666 = call "integrate 1D array interval - double.vi"("Ave N"=w2836, "Array In"=w2838) -> ("Array Out"=w2837:dbl[])  [unwired: 1 out]
      n1667 = Multiply(x=w2846, y=w2836) -> (x*y=w2839:dbl)
      n1668 = Divide(x=w2837, y=w2843) -> (x/y=w2844:dbl[])
      n1669 = Bundle By Name("t0"=w2835, "Y"=w2844, "dt"=w2839) -> (w2845:waveform(dbl))  [unwired: 1 out]
      n1670 = Set Waveform Attribute(5:w2840, 6:w2841, 7:w2845) -> (3:w2842:waveform(dbl))  [unwired: 1 in, 2 out]
    }
    "APD Display Period (s)" <- w2382
    n1671 = Reciprocal(x=w2382) -> (1/x=→"APD Display Freq. (Hz)":dbl)
    n1672 = local read "Display Period (s)"() -> (w2265:dbl)
    n1673 = Increment(x=w2367) -> (x+1=w2368:dbl)
    n1674 = Index Array(array=w2156, index=0) -> (element=w2154:waveform(dbl))
    n1675 = To Double Precision Float(number=w2281) -> (double precision float=w2280:dbl[])
    n1676 = feedback #2(w2368) -> (w2371:dbl)
    n1677 = Select(t=0, s=w2358, f=w2371) -> (s? t:f=w2364:dbl)
    n1678 = Array Size(array=w2280) -> (size(s)=w2370:i32)
    n1679 = Add(x=w2370, y=w2364) -> (x+y=w2365:dbl)
    n1680 = Unbundle By Name(w2154) -> ("Y"=w2152:dbl[])
    n1681 = feedback #3(w2281) -> (w2354:u32[])
    n1682 = Build Array (concatenate)(w2354, w2281) -> (w2351:u32[])
    n1683 = feedback #4(w2217) -> (w2236:u32[])
    n1684 = Divide(x="Bead Sep. Int. Time (s)", y=w2265) -> (x/y=w2150:dbl)
    n1685 = Build Array (concatenate)(w2236, w2217) -> (w2235:u32[])
    n1686 = Greater?(x=w2365, y=w2367) -> (0:w2366:bool)
    n1687 = feedback #5(w2152) -> (w2153:dbl[])
    n1688 = Build Array (concatenate)(w2152, w2153) -> (w2151:dbl[])
    n1689 = Select(t=w2364, s=w2366, f=w2365) -> (s? t:f=w2363:dbl)
    n1690 = feedback-in #2(w2363) -> ()
    n1691 = Array Size(array=w2351) -> (size(s)=w2348:i32)
    n1692 = Array Size(array=w2281) -> (size(s)=w2350:i32)
    n1693 = local read "MCL Scanning"() -> (w2361:bool)
    n1694 = local read "APD Integration Time (s)"() -> (w2244:dbl)
    n1695 = Build Array (concatenate)(w2237, w2387) -> (w2239:waveform(dbl)[])
    "All Signals" <- w2239
    n1696 = Split 1D Array(array=w2151, index=w2150) -> (first subarray=w2144:dbl[])  [unwired: 1 out]
    n1697 = feedback-in #5(w2144) -> ()
    n1698 = Multiply(x=w2350, y="APD Ave N") -> (x*y=w2349:dbl)
    n1699 = Greater?(x=w2348, y=w2349) -> (0:w2352:bool)
    n1700 = Not(x=w2366) -> (.not. x?=w2360:bool)
    n1701 = To Double Precision Float(number=w2217) -> (double precision float=w2216:dbl[])
    n1702 = call-poly <vilib>:"Mean.vi"("X"=w2144) -> ("mean"=w2143:dbl)  [unwired: 1 out]
    "Mean T1 Position (nm)" <- w2143
    n1703 = Subtract(x=w2144, y=w2143) -> (x-y=w2149:dbl[])
    n1704 = Square(x=w2149) -> (x^2=w2148:dbl[])
    n1705 = And(x=w2360, y=w2361) -> (x .and. y?=w2362:bool)
    n1706 = call-poly <vilib>:"Mean.vi"("X"=w2148) -> ("mean"=w2147:dbl)  [unwired: 1 out]
    n1707 = case shown="True" w2352 {
      tunnel: w2351 -> [w2619 w2626]
      tunnel: [w2619 w2624] -> w2297
      tunnel: w2349 -> [_ w2621]
      tunnel: w2348 -> [_ w2625]
      tunnel: w2235 -> [w2618 w2623]
      tunnel: [w2618 w2620] -> w2232
      frame False {
      }
      frame True {
        n1708 = Subtract(x=w2625, y=w2621) -> (x-y=w2622:dbl)
        n1709 = Array Subset(array=w2626, index=w2622, length=w2621) -> (w2624:u32[])
        n1710 = Array Subset(array=w2623, index=w2622, length=w2621) -> (w2620:u32[])
      }
    }
    n1711 = feedback-in #3(w2297) -> ()
    n1712 = feedback-in #4(w2232) -> ()
    n1713 = Or(x=w2362, y=w2358) -> (x .or. y?=w2359:bool)
    n1714 = Square Root(x=w2147) -> (sqrt(x)=w2146:dbl)
    n1715 = Equal?(x="Tab Control 6", y=T36."High Res Display") -> (x = y?=w2287:bool)
    n1716 = Multiply(x="APD Disp. Scale", y=w2237) -> (x*y=w2246:waveform(dbl)[])
    n1717 = Multiply(x="APD Disp. Downsample", y=w2244) -> (x*y=w2242:dbl)
    n1718 = Multiply(x=10.0, y=w2146) -> (x*y=→"Trap 1 Position RMS (A)":dbl)
    n1719 = Divide(x=w2246, y=w2242) -> (x/y=w2214:waveform(dbl)[])
    n1720 = Index Array(array=w2214, index=0) -> (element=w2224:waveform(dbl))
    n1721 = case "For computing FFTs for display" shown="True" "Compute FFT" {
      tunnel: w2241 -> [_ w3296]
      frame False {
      }
      frame True {
        n1722 = Build Array("FFT 1 Choice 1", "FFT 1 Choice 2", "FFT 2 Choice 1", "FFT 2 Choice 2") -> (w3289:u16[])
        n1723 = Array Size(array=w3296) -> (size(s)=w3295:i32)
        n1724 = feedback-in #6(w3289) -> ()
        n1725 = feedback #6(u16[] [100, 100, 100, 100]) -> (w3290:u16[])
        n1726 = feedback-in #7("# Spectra to Ave.") -> ()
        n1727 = feedback #7("# Spectra to Ave.") -> (w3287:dbl)
        n1728 = Not Equal?(x="# Spectra to Ave.", y=w3287) -> (x != y?=w3286:bool)
        n1729 = Not Equal?(x=w3289, y=w3290) -> (x != y?=w3288:bool)
        n1730 = feedback #8(1.0) -> (w3273:dbl)
        n1731 = Compound Arithmetic op=OR("Reset FFT", w3288, w3286) -> (w3271:bool)
        n1732 = Select(t=1.0, s=w3271, f=w3273) -> (s? t:f=w3275:dbl)
        n1733 = Greater?(x=w3275, y="# Spectra to Ave.") -> (0:w3294:bool)
        n1734 = Increment(x=w3275) -> (x+1=w3274:dbl)
        n1735 = feedback-in #8(w3274) -> ()
        n1736 = local read "DMA Update Period (s)"() -> (w3269:dbl)
        n1737 = Multiply(x="# Spectra to Ave.", y=w3269) -> (x*y=→"Ave. Time (s)":dbl)
        n1738 = Build Array(cluster{"f0":dbl, "df":dbl, "magnitude":dbl[]} {"f0"=0.0, "df"=0.0, "magnitude"=[]} ("PSD")) -> (w3278:cluster{"f0":dbl, "df":dbl, "magnitude":dbl[]}[])
        n1739 = Build Array(w3278, w3278, w3278, w3278) -> (w3280:T47)
        n1740 = feedback #9(w3280) -> (w3285:T47)
        n1741 = for {
          N: 4 -> [_]
          tunnel: w3289 -> [w3318] mode=indexing
          tunnel: w3296 -> [w3319]
          tunnel: w3295 -> [w3321]
          tunnel: w3271 -> [w3314]
          tunnel: w3294 -> [w3313]
          tunnel: "# Spectra to Ave." -> [w3312]
          tunnel: [w3311] -> w3284 mode=indexing
          tunnel: w3285 -> [w3316] mode=indexing
          tunnel: [w3315] -> w3272 mode=indexing
          tunnel: w3275 -> [w3310]
          n1742 = Less?(x=w3318, y=w3321) -> (x < y?=w3320:bool)
          n1743 = Index Array(array=w3319, index=w3318) -> (element=w3317:waveform(dbl))
          n1744 = case shown="True" w3320 {
            tunnel: w3317 -> [_ w3338]
            tunnel: w3316 -> [w3323 w3336]
            tunnel: [w3323 w3324] -> w3315
            tunnel: w3314 -> [_ w3335]
            tunnel: w3313 -> [_ w3328]
            tunnel: w3312 -> [_ w3327]
            tunnel: [cluster{"f0":dbl, "df":dbl, "magnitude":dbl[]} {"f0"=0.0, "df"=0.0, "magnitude"=[]} ("PSD") w3329] -> w3311
            tunnel: w3310 -> [_ w3326]
            frame False {
            }
            frame True {
              n1745 = call <vilib>:"Std Deviation and Variance.vi"("X"=w3338) -> ("mean"=w3339:dbl)  [unwired: 1 in, 2 out]
              n1746 = Subtract(x=w3338, y=w3339) -> (x-y=w3337:waveform(dbl))
              n1747 = xnode "Spectral Measurements"("Signals"=w3337) -> ("PSD"=w3331:cluster{"f0":dbl, "df":dbl, "magnitude":dbl[]})  [unwired: 1 in, 1 out]
              n1748 = case shown="False" w3335 {
                tunnel: w3336 -> [w3348 _]
                tunnel: [w3344 w3353] -> w3324
                tunnel: w3331 -> [w3347 w3354]
                tunnel: w3328 -> [w3346 _]
                frame False {
                  n1749 = Build Array (concatenate)(w3348, w3347) -> (w3345:cluster{"f0":dbl, "df":dbl, "magnitude":dbl[]}[])
                  n1750 = case shown="True" w3346 {
                    tunnel: w3345 -> [w3349 w3352]
                    tunnel: [w3349 w3350] -> w3344
                    frame False {
                    }
                    frame True {
                      n1751 = Delete From Array(array=w3352, index=0) -> (array with subset deleted=w3350:cluster{"f0":dbl, "df":dbl, "magnitude":dbl[]}[])  [unwired: 1 in, 1 out]
                    }
                  }
                }
                frame True {
                  n1752 = Build Array(w3354) -> (w3353:cluster{"f0":dbl, "df":dbl, "magnitude":dbl[]}[])
                }
              }
              n1753 = for {
                tunnel: w3324 -> [w3343] mode=indexing
                tunnel: [w3342] -> w3334 mode=indexing
                workers-P: _ -> [_]
                n1754 = Unbundle By Name(w3343) -> ("magnitude"=w3342:dbl[])
              }
              n1755 = Transpose 2D Array(2D array=w3334) -> (transposed array=w3333:dbl[][])
              n1756 = for {
                tunnel: w3333 -> [w3341] mode=indexing
                tunnel: [w3340] -> w3332 mode=indexing
                workers-P: _ -> [_]
                n1757 = Add Array Elements(numeric array=w3341) -> (sum=w3340:dbl)
              }
              n1758 = Select(t=w3327, s=w3328, f=w3326) -> (s? t:f=w3325:dbl)
              n1759 = Divide(x=w3332, y=w3325) -> (x/y=w3330:dbl[])
              n1760 = Bundle By Name(cluster=w3331, "magnitude"=w3330) -> (w3329:cluster{"f0":dbl, "df":dbl, "magnitude":dbl[]})
            }
          }
        }
        n1761 = case shown="True" w3271 {
          tunnel: w3272 -> [w3303 w3309]
          tunnel: [w3303 w3304] -> w3270
          frame False {
          }
          frame True {
            n1762 = Array Subset(array=w3309, index (row)=0 ("index"), length (row)=4 ("length"), index (col)=0 ("index"), length (col)=1 ("length")) -> (w3304:T47)
          }
        }
        n1763 = feedback-in #9(w3270) -> ()
        n1764 = Split 1D Array(array=w3284, index=2) -> (first subarray=→"FFT 1":cluster{"f0":dbl, "df":dbl, "magnitude":dbl[]}[], second subarray=→"FFT 2":cluster{"f0":dbl, "df":dbl, "magnitude":dbl[]}[])
      }
    }
    n1765 = Index Array(array=w2214, index=1) -> (element=w2222:waveform(dbl))
    n1766 = case "For displaying the high resolution display (no downsampling)" shown="True" w2287 {
      tunnel: w2241 -> [_ w2519]
      frame False {
      }
      frame True {
        n1767 = Index Array(array=w2519, index="High Res. Display") -> (element=w2520:waveform(dbl))
        n1768 = call <vilib>:"Std Deviation and Variance.vi"("X"=w2520) -> ("mean"=w2527:dbl, "standard deviation"=w2532:dbl)  [unwired: 1 in, 1 out]
        "Mean Intensity" <- w2527
        "Sigma" <- w2532
        n1769 = Subtract(x=w2520, y=w2527) -> (x-y=w2526:waveform(dbl))
        n1770 = Select(t=w2526, s="Subtract mean", f=w2520) -> (s? t:f=→"1 Channel":waveform(dbl))
        n1771 = Divide(x=w2532, y=w2527) -> (x/y=→"Sigma/Mean":dbl)
        n1772 = feedback #10(1) -> (w2521:i32)
        n1773 = Greater Or Equal?(x=w2521, y="Slow mean N ave.") -> (x >= y?=w2534:bool)
        n1774 = Increment(x=w2521) -> (x+1=w2536:i32)
        n1775 = Select(t=1, s=w2534, f=w2536) -> (s? t:f=w2523:i32)
        n1776 = feedback-in #10(w2523) -> ()
        n1777 = feedback #11() -> (w2524:waveform(dbl))  [unwired: 1 out]
        n1778 = case shown="Default" w2521 {
          tunnel: [w2539 w2542] -> w2525
          tunnel: w2524 -> [w2541 _]
          tunnel: w2520 -> [w2540 w2542]
          frame Default {
            n1779 = call-poly <vilib>:"Append Waveforms.vi"("waveform B"=w2540, "waveform A"=w2541) -> ("waveform out"=w2539:waveform(dbl))  [unwired: 1 in, 8 out]
          }
          frame 1 {
          }
        }
        n1780 = feedback-in #11(w2525) -> ()
        n1781 = case shown="True" w2534 {
          tunnel: w2525 -> [_ w2538]
          frame False {
          }
          frame True {
            n1782 = call-poly <vilib>:"Mean.vi"("X"=w2538) -> ("mean"=→"Slow mean":dbl)  [unwired: 1 out]
          }
        }
      }
    }
    n1783 = case "For plotting results of scanning MCL" shown="True" w2359 {
      tunnel: w2358 -> [_ w2659]
      tunnel: w2280 -> [_ w2755]
      tunnel: w2367 -> [_ _]
      tunnel: w2241 -> [_ w2729]
      tunnel: w2216 -> [_ w2660]
      tunnel: w2215 -> [_ w2633]
      frame False {
      }
      frame True {
        w2640 = u32 0 items=["Horizontal", "Vertical", "Central", "1st Diagonal", "2nd Diagonal"] ("Type of Symmetry")
        w2668 = u32 0 items=["Horizontal", "Vertical", "Central", "1st Diagonal", "2nd Diagonal"] ("Type of Symmetry")
        w2671 = u32 0 items=["Horizontal", "Vertical", "Central", "1st Diagonal", "2nd Diagonal"] ("Type of Symmetry")
        w2700 = u32 0 items=["Horizontal", "Vertical", "Central", "1st Diagonal", "2nd Diagonal"] ("Type of Symmetry")
        n1784 = Index Array(array=w2729, index=10) -> (element=w2735:waveform(dbl))
        n1785 = Index Array(array=w2729, index=11) -> (element=w2732:waveform(dbl))
        n1786 = local read "Cycles/step (MCL)"() -> (w2685:u64)
        n1787 = Index Array(array=w2729, index="Channel") -> (element=w2731:waveform(dbl))
        n1788 = Unbundle(w2633) -> ("New Image"=w2632:T3, "New Image"=w2631:T3, "New Image"=w2630:T3, "New Image"=w2629:T3)
        n1789 = Unbundle By Name(w2735) -> ("Y"=w2687:dbl[])
        n1790 = Unbundle By Name(w2732) -> ("Y"=w2689:dbl[])
        n1791 = Unbundle By Name(w2731) -> ("Y"=w2694:dbl[])
        n1792 = call "downsample 1D array - double.vi"("Ave N"=w2685, "Array In"=w2687) -> ("Array Out"=w2686:dbl[])  [unwired: 1 out]
        n1793 = call "downsample 1D array - double.vi"("Ave N"=w2685, "Array In"=w2689) -> ("Array Out"=w2688:dbl[])  [unwired: 1 out]
        n1794 = call "downsample 1D array - double.vi"("Ave N"=w2685, "Array In"=w2694) -> ("Array Out"=w2693:dbl[])  [unwired: 1 out]
        n1795 = feedback #12(w2755) -> (w2756:dbl[])
        n1796 = Build Array (concatenate)(w2756, w2755) -> (w2737:dbl[])
        n1797 = feedback #13(w2660) -> (w2662:dbl[])
        n1798 = Build Array (concatenate)(w2662, w2660) -> (w2661:dbl[])
        n1799 = local read "Scan steps (MCL)"() -> (w2642:u64)
        n1800 = Select(t=w2755, s=w2659, f=w2737) -> (s? t:f=w2741:dbl[])
        n1801 = feedback-in #12(w2741) -> ()
        n1802 = Select(t=w2660, s=w2659, f=w2661) -> (s? t:f=w2643:dbl[])
        n1803 = feedback-in #13(w2643) -> ()
        n1804 = local read "Scan lines (y)"() -> (w2628:u64)
        n1805 = local read "N APD Samp/step"() -> (w2644:dbl)
        n1806 = feedback #14(w2686) -> (w2743:dbl[])
        n1807 = Build Array (concatenate)(w2743, w2686) -> (w2734:dbl[])
        n1808 = feedback #15(w2693) -> (w2753:dbl[])
        n1809 = Build Array (concatenate)(w2753, w2693) -> (w2752:dbl[])
        n1810 = feedback #16(w2688) -> (w2745:dbl[])
        n1811 = Build Array (concatenate)(w2745, w2688) -> (w2746:dbl[])
        n1812 = Select(t=w2686, s=w2659, f=w2734) -> (s? t:f=w2690:dbl[])
        n1813 = feedback-in #14(w2690) -> ()
        n1814 = Select(t=w2693, s=w2659, f=w2752) -> (s? t:f=w2692:dbl[])
        n1815 = feedback-in #15(w2692) -> ()
        n1816 = Select(t=w2688, s=w2659, f=w2746) -> (s? t:f=w2691:dbl[])
        n1817 = feedback-in #16(w2691) -> ()
        n1818 = Multiply(x=w2642, y=u64 2) -> (x*y=w2627:u64)
        n1819 = call "integrate 1D array interval - double.vi"("Ave N"=w2644, "Array In"=w2643) -> ("Array Out"=w2655:dbl[])  [unwired: 1 out]
        n1820 = call "integrate 1D array interval - double.vi"("Ave N"=w2644, "Array In"=w2741) -> ("Array Out"=w2740:dbl[])  [unwired: 1 out]
        n1821 = Array Size(array=w2655) -> (size(s)=w2656:i32)
        n1822 = Array Size(array=w2740) -> (size(s)=w2742:i32)
        n1823 = Multiply(x=w2628, y=w2627) -> (x*y=w2658:u64)
        n1824 = Multiply(x=w2628, y=w2627) -> (x*y=w2750:u64)
        n1825 = call-poly <vilib>:"Mean.vi"("X"=w2690) -> ("mean"=w2674:dbl)  [unwired: 1 out]
        n1826 = Subtract(x=w2658, y=w2656) -> (x-y=w2649:u64)
        n1827 = call-poly <vilib>:"Mean.vi"("X"=w2692) -> ("mean"=w2679:dbl)  [unwired: 1 out]
        n1828 = call-poly <vilib>:"Mean.vi"("X"=w2691) -> ("mean"=w2677:dbl)  [unwired: 1 out]
        n1829 = call-poly <vilib>:"Mean.vi"("X"=w2655) -> ("mean"=w2646:dbl)  [unwired: 1 out]
        n1830 = Subtract(x=w2750, y=w2742) -> (x-y=w2684:u64)
        n1831 = call-poly <vilib>:"Mean.vi"("X"=w2740) -> ("mean"=w2681:dbl)  [unwired: 1 out]
        n1832 = Initialize Array(1.0 ("element"), w2649) -> (w2645:dbl[])
        n1833 = Initialize Array(1.0 ("element"), w2684) -> (w2675:dbl[])
        n1834 = Multiply(x=w2645, y=w2646) -> (x*y=w2647:dbl[])
        n1835 = Multiply(x=w2675, y=w2677) -> (x*y=w2678:dbl[])
        n1836 = Multiply(x=w2675, y=w2679) -> (x*y=w2680:dbl[])
        n1837 = Multiply(x=w2675, y=w2674) -> (x*y=w2676:dbl[])
        n1838 = Multiply(x=w2675, y=w2681) -> (x*y=w2682:dbl[])
        n1839 = Build Array (concatenate)(w2690, w2676) -> (w2744:dbl[])
        n1840 = Build Array (concatenate)(w2692, w2680) -> (w2748:dbl[])
        n1841 = Build Array (concatenate)(w2691, w2678) -> (w2747:dbl[])
        n1842 = Build Array (concatenate)(w2655, w2647) -> (w2657:dbl[])
        n1843 = Build Array (concatenate)(w2740, w2682) -> (w2749:dbl[])
        n1844 = Reshape Array(w2744, w2628, w2627) -> (w2710:dbl[][])
        n1845 = Reshape Array(w2657, w2628, w2627) -> (w2653:dbl[][])
        n1846 = Reshape Array(w2748, w2628, w2627) -> (w2702:dbl[][])
        n1847 = Reshape Array(w2747, w2628, w2627) -> (w2717:dbl[][])
        n1848 = Reshape Array(w2749, w2628, w2627) -> (w2727:dbl[][])
        n1849 = Array Subset(array=w2717, index (col)=0 ("index"), length (col)=w2642) -> (w2722:dbl[][])  [unwired: 2 in]
        n1850 = Array Subset(array=w2717, index (col)=w2642) -> (w2720:dbl[][])  [unwired: 3 in]
        n1851 = Array Subset(array=w2702, index (col)=0 ("index"), length (col)=w2642) -> (w2708:dbl[][])  [unwired: 2 in]
        n1852 = Array Subset(array=w2702, index (col)=w2642) -> (w2706:dbl[][])  [unwired: 3 in]
